vi "EncodeLVImageToBase64.vi"(7 "Compression (none)":i32, 8 "error in (no error)":errorcluster, 11 "LVImage":T1) -> (0 "error out":errorcluster, 3 "Base64String":string)   [LabVIEW 2020]
doc: "Encode a LabView Image to a Base64 Data URI"
uses:
  <vilib>/picture/picture.llb/imagedata.ctl
  <vilib>/wsapi/NI_WebServices.lvlib
  <vilib>/JDP Science/JDP Science Common Utilities/Base64/Base64 Support.lvlib
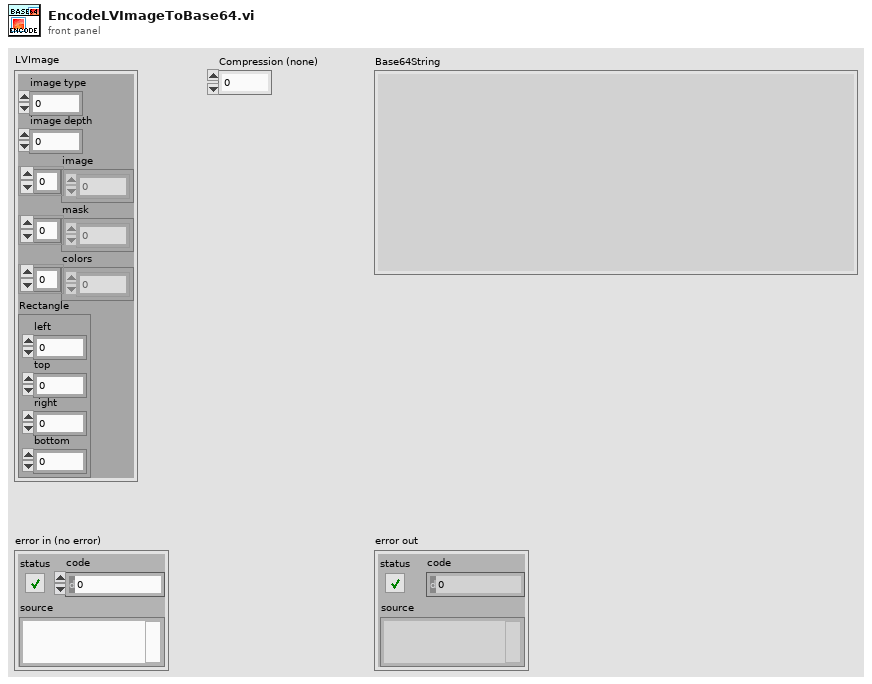
[diagram p1: front panel]
types:
  T1 = typedef "imagedata.ctl" = cluster{"image type":i32, "image depth":i32, "image":u8[], "mask":u8[], "colors":u32[], "Rectangle":cluster{"left":i16, "top":i16, "right":i16, "bottom":i16}}
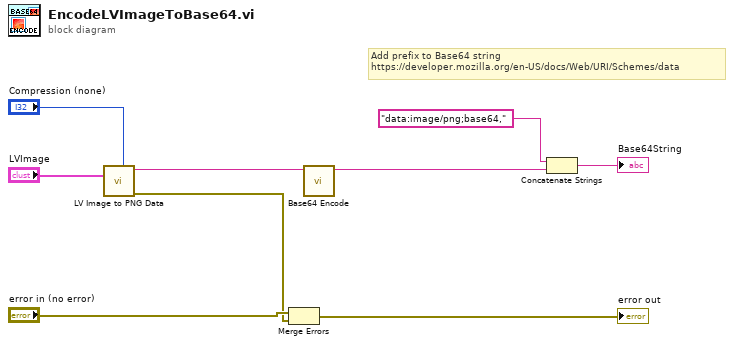
[diagram p0: block diagram]
diagram:
  # "Add prefix to Base64 string\nhttps://developer.mozilla.org/en-US/docs/Web/URI/Schemes/data"
  n1 = call <vilib>:"LV Image to PNG Data.vi"("compression (none)"="Compression (none)", "image data"="LVImage") -> ("error out"=w5:errorcluster, "png data"=w9:string)  [unwired: 8 in]
  n2 = Merge Errors("error in (no error)", w5) -> (→"error out":errorcluster)
  n3 = call <vilib>:"Base64 Encode.vi"("String to Encode"=w9) -> ("Base64 Encoded"=w3:string)  [unwired: 10 in]
  n4 = Concatenate Strings("data:image/png;base64,", w3) -> (→"Base64String":string)
